vi "Init.vi"(3 "Container State":T4, 4 "Previous State":variant, 5 "Previous Version":T3) -> (2 "Current State":T1)   [LabVIEW 2020, in "2D Error Bar.xctl"]
uses:
  <vilib>/Math Plots/2D Math Plots/2D Error Bar/2D Error Bar XCtrl/2D Error Bar.xctl
  <vilib>/Math Plots/2D Math Plots/2D Error Bar/2D Error Bar XCtrl/State.ctl
  <vilib>/Math Plots/2D Math Plots/2D Error Bar/2D Error Bar/2D Error Bar.lvclass
  <vilib>/Math Plots/2D Math Plots/2D Plot/Action String/2DMathPlot Ctrl Act Queue.ctl
  <vilib>/Math Plots/2D Math Plots/2D Plot/Action String/2DMathPlot Ctrl Act Cluster.ctl
  <vilib>/Math Plots/2D Math Plots/2D Plot/Action String/2DMathPlot State Class.ctl
  <vilib>/_xctls/Container State.ctl
  <vilib>/_xctls/Version.ctl
  <vilib>/_xctls/XControlSupport.lvlib
panel:
  in  "Default Indicator State":T1={"2D Error Bar.lvclass"=refnum, "Control Ref Queue"=refnum, "Main Frame Color"=12369084, "Plot Legend Color"=12369084}
  in  "Default Control State":T1={"2D Error Bar.lvclass"=refnum, "Control Ref Queue"=refnum, "Main Frame Color"=12369084, "Plot Legend Color"=12369084}
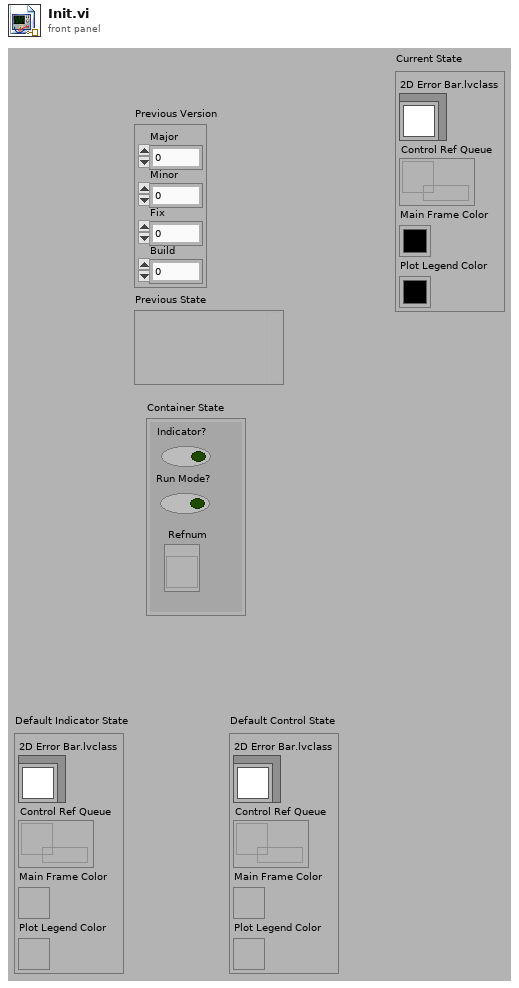
[diagram p1: front panel]
types:
  T1 = typedef "2D Error Bar.xctl/State.ctl" = cluster{"2D Error Bar.lvclass":refnum<class "2D Error Bar.lvclass">, "Control Ref Queue":T2, "Main Frame Color":u32, "Plot Legend Color":u32}
  T2 = typedef "2DMathPlot Ctrl Act Queue.ctl" = refnum<queue>
  T3 = typedef "XControlSupport.lvlib/Version.ctl" = cluster{"Major":u16, "Minor":u16, "Fix":u16, "Build":u16}
  T4 = typedef "XControlSupport.lvlib/Container State.ctl" = cluster{"Indicator?":bool, "Run Mode?":bool, " Refnum":refnum<vi>}
  T5 = typedef "2DMathPlot Ctrl Act Cluster.ctl" = cluster{"Plot Area Ref":refnum<vi>, "Z Axis Ref":refnum<vi>, "Legend Ref":refnum<vi>, "XControl Ref":refnum<vi>, "Facade Ref":refnum<vi>, "Display State Change Class":T6}
  T6 = typedef "2DMathPlot State Class.ctl" = enum16{"Update All (Undo)", "Update General", "Update Appearance", "Update Format", "Update Scale", "Update Marker", "Update Cursor", "None"}
  T7 = cluster{"2D Error Bar.lvclass":refnum<class "2D Error Bar.lvclass">, "Control Ref Queue":T2}
  T8 = cluster{"2D Error Bar.lvclass":refnum<class "2D Error Bar.lvclass">, "Control Ref Queue":T2, "Frame Color":u32, "Frame Color":u32}
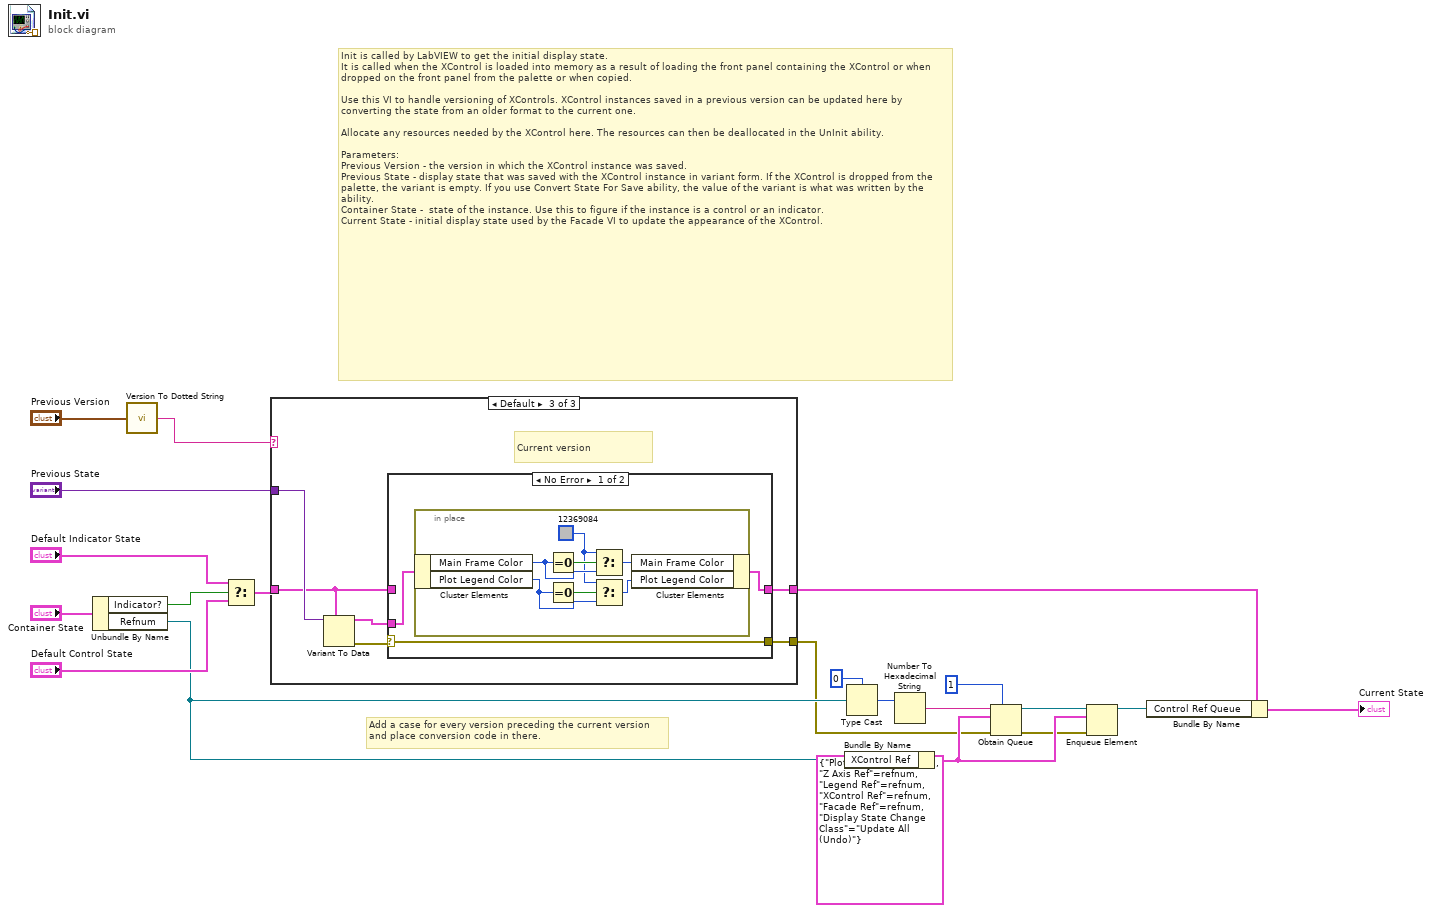
[diagram p0: block diagram]
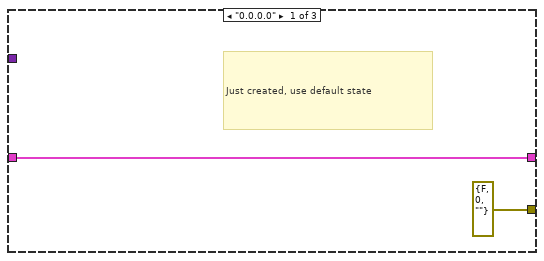
[diagram p2: hidden frame]
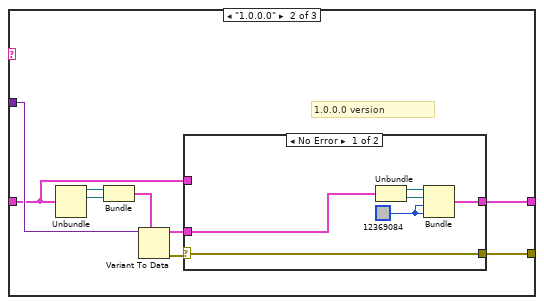
[diagram p3: hidden frame]
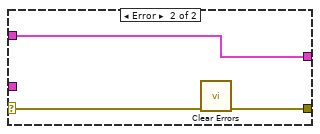
[diagram p4: hidden frame]
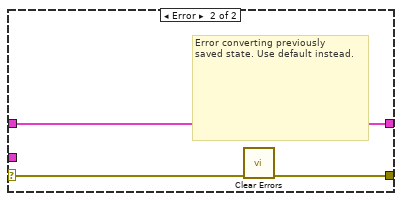
[diagram p5: hidden frame]
diagram:
  # "Add a case for every version preceding the current version and place conversion code in there."
  # "Init is called by LabVIEW to get the initial display state.\nIt is called when the XControl is loaded into memory as a result of loading the front panel containing the XControl or when dropped on the front panel from the palette or when copied.\n\nUse this VI to handle versioning of XControls. XControl instances saved in a previous version can be updated here by converting the state from an older format to the current one.\n\nAllocate any resources needed by the XControl here. The resources can then be deallocated in the UnInit ability.\n\nParameters:\nPrevious Version - the version in which the XControl instance was saved.\nPrevious State - display state that was saved with the XControl instance in variant form. If the XControl is dropped from the palette, the variant is empty. If you use Convert State For Save ability, the value of the variant is what was written by the ability. \nContainer State -  state of the instance. Use this to figure if the instance is a control or an indicator.\nCurrent State - initial display state used by the Facade VI to update the appearance of the XControl."
  n1 = Unbundle By Name("Container State") -> ("Indicator?"=w17:bool, "Refnum"=w4:refnum<vi>)
  n2 = call <vilib>:"Version To Dotted String.vi"("Version"="Previous Version") -> ("String Version"=w14:string)
  n3 = Select(t="Default Indicator State", s=w17, f="Default Control State") -> (s? t:f=w16:T1)
  n4 = case shown="Default" w14 {
    tunnel: "Previous State" -> [_ w27 w47]
    tunnel: [w23 w25 w43] -> w3
    tunnel: w16 -> [w23 w26 w44]
    tunnel: [errorcluster {"status"=FALSE, "code"=0, "source"=""} ("error IO") w24 w42] -> w1
    frame "0.0.0.0" {
      # "Just created, use default state"
    }
    frame "1.0.0.0" {
      # "1.0.0.0 version"
      n5 = Unbundle(w26) -> ("2D Error Bar.lvclass"=w31:refnum<class "2D Error Bar.lvclass">, "Control Ref Queue"=w32:T2)  [unwired: 2 out]
      n6 = Bundle("2D Error Bar.lvclass"=w31, "Control Ref Queue"=w32) -> (w30:T7)  [unwired: 1 in]
      n7 = Variant To Data(type=w30, Variant=w27) -> (data=w29:T7, error out=w28:errorcluster)  [unwired: 1 in]
      n8 = case shown="No Error" w28 {
        selector: w28 -> [w38 w40]
        tunnel: w29 -> [w36 _]
        tunnel: [w34 w41] -> w25
        tunnel: w26 -> [_ w41]
        tunnel: [w38 w39] -> w24
        frame No Error {
          w33 = u32 12369084 ("Frame Color")
          n9 = Unbundle(w36) -> ("2D Error Bar.lvclass"=w37:refnum<class "2D Error Bar.lvclass">, "Control Ref Queue"=w35:T2)
          n10 = Bundle("2D Error Bar.lvclass"=w37, "Control Ref Queue"=w35, "Frame Color"=w33, "Frame Color"=w33) -> (w34:T8)  [unwired: 1 in]
        }
        frame Error {
          n11 = call <vilib>:"Clear Errors.vi"("error in (no error)"=w40) -> ("error out"=w39:errorcluster)  [unwired: 1 in, 5 out]
        }
      }
    }
    frame Default {
      # "Current version"
      n12 = Variant To Data(type=w44, Variant=w47) -> (data=w45:T1, error out=w46:errorcluster)  [unwired: 1 in]
      n13 = case shown="No Error" w46 {
        selector: w46 -> [w50 w59]
        tunnel: w45 -> [w49 _]
        tunnel: [w48 w60] -> w43
        tunnel: w44 -> [_ w60]
        tunnel: [w50 w58] -> w42
        frame No Error {
          n14 = in-place {
            w51 = u32 12369084 ("Frame Color")
            n15 = in-place-cluster #1(w49) -> ("Main Frame Color"=w55:u32, "Plot Legend Color"=w53:u32)
            n16 = Equal To 0?(x=w55) -> (x = 0?=w57:bool)
            n17 = Equal To 0?(x=w53) -> (x = 0?=w54:bool)
            n18 = Select(t=w51, s=w57, f=w55) -> (s? t:f=w56:u32)
            n19 = Select(t=w51, s=w54, f=w53) -> (s? t:f=w52:u32)
            n20 = in-place-cluster #1("Main Frame Color"=w56, "Plot Legend Color"=w52) -> (w48:T1)
          }
        }
        frame Error {
          # "Error converting previously \nsaved state. Use default instead."
          n21 = call <vilib>:"Clear Errors.vi"("error in (no error)"=w59) -> ("error out"=w58:errorcluster)  [unwired: 1 in, 5 out]
        }
      }
    }
  }
  n22 = Bundle By Name(cluster=T5 {"Plot Area Ref"=refnum, "Z Axis Ref"=refnum, "Legend Ref"=refnum, "XControl Ref"=refnum, "Facade Ref"=refnum, "Display State Change Class"=enum."Update All (Undo)"} ("Control Ref Cluster"), "XControl Ref"=w4) -> (w7:T5)
  n23 = Type Cast(type=u64 0, x=w4) -> (*(type *) &x=w13:u64)
  n24 = Number To Hexadecimal String(2:w13) -> (0:w11:string)  [unwired: 1 out]
  n25 = Obtain Queue(max queue size (-1, unlimited)=1, name (unnamed)=w11, element data type=w7, error in (no error)=w1) -> (queue out=w9:refnum<queue>, error out=w6:errorcluster)  [unwired: 1 in, 1 out]
  n26 = Enqueue Element(queue=w9, element=w7, error in (no error)=w6) -> (queue out=w8:refnum<queue>)  [unwired: 3 out]
  n27 = Bundle By Name(cluster=w3, "Control Ref Queue"=w8) -> (→"Current State":T1)
